vi "FRIC_navX_Get_Registry.vi"(5 "Device Number":T1, 7 "Update":bool, 9 "Connected?":bool, 11 "Registry (in)":u8[](array[numeric])) -> (1 "Connected?":bool, 3 "Registry (out)":u8[](array[numeric]))   [LabVIEW 2016]
uses:
  TypeDefs/FRIC_navX_DeviceNumbersTypeDef.ctl
panel:
  out "Array 2":bool[](array[boolean])
  out "Array":u8[][](array[numeric])
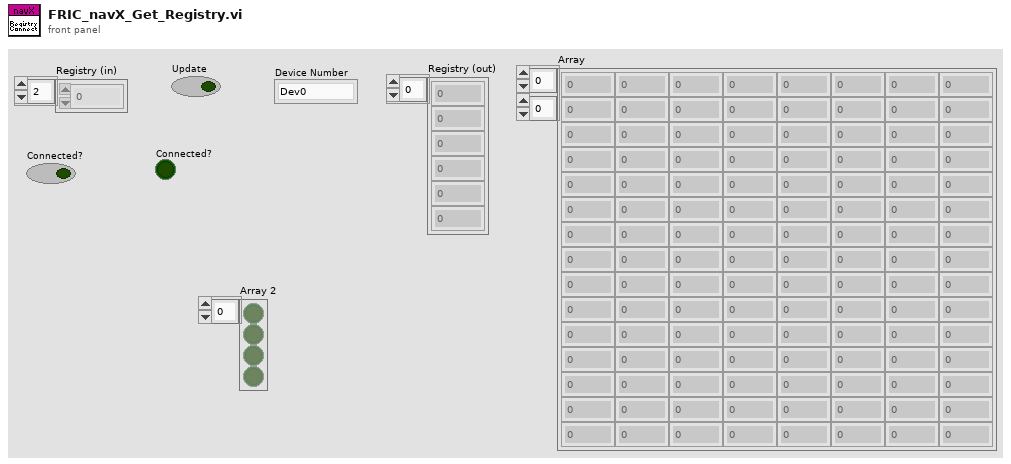
[diagram p1: front panel]
types:
  T1 = typedef "FRIC_navX_DeviceNumbersTypeDef.ctl" = enum16{"Dev0", "Dev1", "Dev2", "Dev3"}
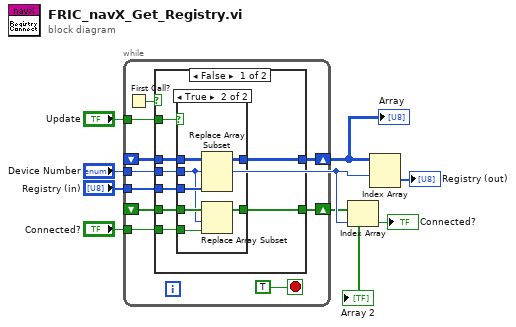
[diagram p0: block diagram]
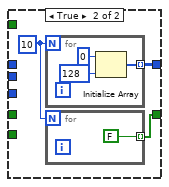
[diagram p3: hidden frame]
diagram:
  n1 = while {
    tunnel: "Update" -> [w17]
    tunnel: "Registry (in)" -> [w16]
    shift-right: [w14] -> w3
    shift-left: _ -> [w13]
    tunnel: "Connected?" -> [w15]
    shift-right: [w10] -> w6
    shift-left: _ -> [w11]
    tunnel: "Device Number" -> [w12]
    stop <- TRUE stop-if-true
    n2 = First Call?() -> (First Call?: T/F=w9:bool)
    n3 = case shown="False" w9 {
      tunnel: w17 -> [w26 _]
      tunnel: w16 -> [w25 _]
      tunnel: w15 -> [w24 _]
      tunnel: [w23 w38] -> w14
      tunnel: w13 -> [w22 _]
      tunnel: w12 -> [w21 _]
      tunnel: w11 -> [w20 _]
      tunnel: [w19 w36] -> w10
      frame False {
        n4 = case shown="True" w26 {
          tunnel: w25 -> [_ w35]
          tunnel: w24 -> [_ w29]
          tunnel: [w28 w31] -> w23
          tunnel: w22 -> [w28 w32]
          tunnel: w21 -> [_ w30]
          tunnel: w20 -> [w27 w34]
          tunnel: [w27 w33] -> w19
          frame False {
          }
          frame True {
            n5 = Replace Array Subset(array=w34, new element=w35, index (row)=w30) -> (w33:u8[][])  [unwired: 1 in]
            n6 = Replace Array Subset(array=w32, new element=w29, index=w30) -> (w31:bool[])
          }
        }
      }
      frame True {
        w37 = 10
        n7 = for {
          N: w37 -> [_]
          tunnel: [w40] -> w36 mode=indexing
          n8 = Initialize Array(u8 0 ("Received Data"), 128 ("hex")) -> (w40:u8[])
        }
        n9 = for {
          N: w37 -> [_]
          tunnel: [FALSE] -> w38 mode=indexing
        }
      }
    }
  }
  "Array" <- w6
  "Array 2" <- w3
  n10 = Index Array(array=w3, index="Device Number") -> (element=→"Connected?":bool)
  n11 = Index Array(array=w6, index (row)="Device Number") -> (element=→"Registry (out)":u8[])  [unwired: 1 in]
